vi "main.vi"() -> ()   [LabVIEW 2016]
uses:
  <vilib>/myRIO/Instrument Drivers/Onboard IO/DIO/typedefs/DIO Reference.ctl
  <vilib>/myRIO/Common/Instrument Driver Framework/Utilities/typedefs/myRIO Generic Hardware Reference.ctl
  <vilib>/myRIO/Common/Instrument Driver Framework/Utilities/typedefs/Hardware Version Enum.ctl
  <vilib>/myRIO/Common/Instrument Driver Framework/Utilities/typedefs/myRIO v1.0 Reference.ctl
  <vilib>/myRIO/Common/Instrument Driver Framework/Utilities/typedefs/Generic FPGA Reference.ctl
  <vilib>/myRIO/Common/Instrument Driver Framework/myRIO v1.0/DIO/typedefs/DIO Channels List.ctl
  <vilib>/myRIO/Common/Instrument Driver Framework/myRIO v1.0/DIO/typedefs/DIO Channels Enum.ctl
  <vilib>/userdefined/High Color/nirio_resource_hc.ctl
  <vilib>/userdefined/High Color/IMAQdx.ctl
  <vilib>/vision/Instrument.llb/QR Code Search Options.ctl
  <vilib>/vision/Instrument.llb/Demodulation Mode.ctl
  <vilib>/vision/Instrument.llb/Cell Sample Size.ctl
  <vilib>/vision/Instrument.llb/Cell Filter Mode.ctl
  <vilib>/vision/driver/IMAQdx.llb/IMAQdx Camera Control Mode.ctl
  <vilib>/myRIO/Common/Instrument Driver Framework/Utilities/vis/Is FPGA Ref Available.vi
  <vilib>/myRIO/Common/Instrument Driver Framework/myRIO v1.0/DIO/vis/myRIO v1.1 Open DIO.vi
  <vilib>/myRIO/Instrument Drivers/Onboard IO/DIO/vis/Write.vi
  <vilib>/myRIO/Instrument Drivers/Onboard IO/DIO/vis/Read.vi
  <vilib>/myRIO/Common/Instrument Driver Framework/Utilities/vis/Validate Channels.vi
  <vilib>/myRIO/Common/Instrument Driver Framework/myRIO v1.0/DIO/vis/myRIO v1.0 Reserve DIO.vi
  <vilib>/myRIO/Common/Instrument Driver Framework/myRIO v1.0/UART/vis/myRIO v1.0 Close UART.vi
  <vilib>/myRIO/Common/Instrument Driver Framework/myRIO v1.0/Resource Manager/vis/myRIO v1.0 Reserve Channel List.vi
  <vilib>/myRIO/Common/Instrument Driver Framework/myRIO v1.0/DIO/vis/myRIO v1.0 Build MUX Configuration DIO.vi
  <vilib>/myRIO/Common/Instrument Driver Framework/myRIO v1.0/Resource Manager/vis/myRIO v1.0 Reserve Channel.vi
  <vilib>/myRIO/Common/Instrument Driver Framework/myRIO v1.0/Resource Manager/vis/myRIO v1.0 Unreserve Channel.vi
  <vilib>/myRIO/Common/Instrument Driver Framework/myRIO v1.0/Resource Manager/vis/myRIO v1.0 Create Configuration List.vi
  <vilib>/myRIO/Common/Instrument Driver Framework/myRIO v1.0/Resource Manager/vis/myRIO v1.0 Build Mutex Name.vi
  <vilib>/Utility/VariantDataType/GetNumericInfo.vi
  <vilib>/Utility/error.llb/Error Cluster From Error Code.vi
  <vilib>/myRIO/Common/Instrument Driver Framework/myRIO v1.0/myRIO v1.1 Open.vi
  <vilib>/myRIO/Common/Instrument Driver Framework/Utilities/vis/IO Manager.vi
  <vilib>/myRIO/Common/Instrument Driver Framework/Utilities/vis/Configuration Manager.vi
  <vilib>/myRIO/Common/Instrument Driver Framework/myRIO v1.0/Resource Manager/vis/myRIO v1.0 Configure IO.vi
  <vilib>/myRIO/Common/Instrument Driver Framework/myRIO v1.0/myRIO v1.0 Close.vi
  <vilib>/myRIO/Common/Instrument Driver Framework/myRIO v1.0/DIO/vis/myRIO v1.0 Write DIO.vi
  <vilib>/myRIO/Common/Instrument Driver Framework/myRIO v1.0/DIO/vis/myRIO v1.0 Read DIO.vi
  <vilib>/Utility/file.llb/Read Delimited Spreadsheet (string).vi
  <vilib>/myRIO/Common/Instrument Driver Framework/Utilities/vis/FPGA Ref Manager.vi
  <vilib>/myRIO/Common/Instrument Driver Framework/myRIO v1.0/myRIO v1.0 Reset FPGA.vi
  <vilib>/myRIO/Common/Instrument Driver Framework/myRIO v1.0/IRQ/vis/myRIO v1.0 IRQ Info FGV.vi
  <vilib>/myRIO/Common/Instrument Driver Framework/myRIO v1.0/IRQ/vis/myRIO v1.0 Timer IRQ Info FGV.vi
  <vilib>/myRIO/Common/Instrument Driver Framework/myRIO v1.0/IRQ/vis/myRIO v1.0 ISR Agent.vi
  <instrlib>/Hokuyo URG Series/Public/Initialize-cRIO-USB.vi
  <vilib>/myRIO/Express VI/Onboard Devices/LED/LED Express VI.xnode
  <vilib>/myRIO/Instrument Drivers/Onboard IO/DIO/vis/myRIO DIO Open.xnode
  <vilib>/myRIO/Express VI/Onboard IO/DI/DI Express VI.xnode
  <vilib>/myRIO/Instrument Drivers/Onboard IO/DIO/DIO.lvlib
  <vilib>/vision/driver/NI_Vision_Acquisition_Software.lvlib
  <vilib>/myRIO/Instrument Drivers/Utilities/Utilities.lvlib
  <instrlib>/Hokuyo URG Series/Hokuyo URG Series.lvlib
  <vilib>/vision/NI_Vision_Development_Module.lvlib
panel:
  out "Color Footage":T1(plugin-control)
  out "QR Footage":T1(plugin-control)
  out "QR Attempts":i32
  out "Data":string
  out "?":errorcluster
  out "Algorithm log":string
  out "Cubes 3 Flag":bool
  out "Delete Files":bool
  out "Hokuyo Init":bool
  out "hokuyo instance":dbl[](array[numeric])
  out "hokuyo":dbl[](array[numeric])
  out "COLOR CUBE":dbl
  out "COLOR BOX":dbl
  out "Box Array":dbl[](array[numeric])
  out "Cube Array":dbl[](array[numeric])
  out "Box Green":dbl
  out "Box Red":dbl
  out "Box Blue":dbl
  out "Cube Green":dbl
  out "Cube Red":dbl
  out "Cube Blue":dbl
  out "Colors String":string
  out "QR BREAK":bool
  out "CHECK route2.csv":bool
  out "Route Size Array":dbl[](array[numeric])
  out "MovementCounter":dbl
  out "ActionCounter":dbl
  out "Route Size":dbl
  out "Action":dbl
  out "Movement":dbl
  out "Route":string[][](array[string])
  out "START ALGO":bool
  out "CHECK route1.csv":bool
  out "TERMINAL OUTPUT":string
  out "STD ERROR":string
  out "RETURN VALUE":i32
  # "+\n+\n+\n+\n+\n+\n+\n+\n+\n+\n+\n+\n+\n+\n+\n+\n+\n+\n+\n+\n+\n+\n+\n+\n+\n+\n+\n+\n+\n+\n+\n+\n+\n+\n+\n+\n+\n+\n+\n+\n+\n+\n+\n+\n+\n+\n+\n+\n+\n+\n+\n+\n+\n+\n+\n+\n+\n+\n+\n+\n+"
  # "+\n+\n+\n+\n+\n+\n+\n+\n+\n+\n+\n+\n+\n+\n+\n+\n+\n+\n+\n+\n+"
  # "++++++++++++++++++++++++++++++++++++++++++++++++++++++++++++++++++++++++++++++++++++++++++++++++++++++++++++++++++++++++++++++++++++++++++++++++++++++++++++++++++++++++++++++++++++++++++++++++++++++++++++++++++++++++++++++++++++++++"
  # "+\n+\n+\n+\n+\n+\n+\n+\n+\n+\n+\n+\n+\n+\n+\n+\n+\n+\n+\n+\n+\n+\n+\n+\n+\n+\n+\n+\n+\n+\n+\n+\n+\n+\n+\n+\n+\n+\n+\n+\n+\n+\n+\n+\n+\n+\n+\n+\n+\n+\n+\n+\n+\n+\n+\n+\n+\n+\n+\n+"
  # "+\n+\n+\n+\n+\n+\n+\n+\n+\n+\n+\n+\n+\n+\n+\n+\n+\n+\n+\n+\n+\n+\n+\n+\n+\n+\n+\n+\n+\n+\n+\n+\n+\n+\n+\n+\n+\n+\n+\n+\n+\n+\n+\n+\n+\n+\n+\n+"
  # "+\n+\n+\n+\n+\n+\n+\n+\n+\n+\n+\n+\n+\n+\n+\n+\n+\n+\n+\n+\n+"
  # "+\n+\n+\n+\n+\n+\n+\n+\n+\n+\n+\n+\n+\n+\n+\n+\n+\n+\n+\n+\n+"
  # "INDICATORS"
  # "QR INDICATOR"
  # "ALGORITHM"
  # "NUMERIC INDICATORS"
  # "INFO"
  # "Actions:\n\n0) Finish\n1) Front\n2) Back\n3) Right\n4) Left\n5) Calibrate\n6) Take and Store\n7) Take and Hold\n8) Place cube\n9) Color Check\n10) Park\n15) No Calibration"
  # "Colors:\n\n10) Blue\n11) Green\n12) Yellow\n13) Red\n14) Orange\n15) Unknown"
  # "++++++++++++++++++++++++++++++++++++++++++++++++++++++++++++++++++++++++++++++++++++++++++++++++++++++++++++++++++++++++++++++++++++++++++++++++++++++++++++++++++++++++++++++++++++++++++++++++++++++++++++++++++++++++++++++++++++++"
  # "+\n+\n+\n+\n+\n+\n+\n+\n+\n+\n+\n+\n+\n+\n+\n+\n+\n+\n+\n+\n+\n+\n+\n+\n+\n+"
  # "+\n+\n+\n+\n+\n+\n+\n+\n+\n+\n+\n+\n+\n+\n+\n+\n+\n+\n+\n+\n+\n+\n+\n+\n+\n+\n+\n+\n+\n+\n+\n+\n+\n+\n+\n+\n+\n+"
  # "BASH CLEANUP SCRIPT"
  # "ROUTE FILES CHECK"
  # "ROUTE READING"
  # "++++++++++++++++++++++++++++++++++++++++++++++++++++++++++++++++++++++++++++++++++++++++++++++++++++++++++++++++"
  # "HOKUYO CALIBRATION"
  # "10"
  # "11"
  # "++++++++++++++++++++++++++++++++++++++++++++++++++++++++++++++++++++++++++++++++++++++++++++++++++++++++++++++++++++++++++++++++++++++++++++++++++++++++++++++++++++++++++++++++++++++++++++++++++++++++++++++++++++++++++++++++++++++++"
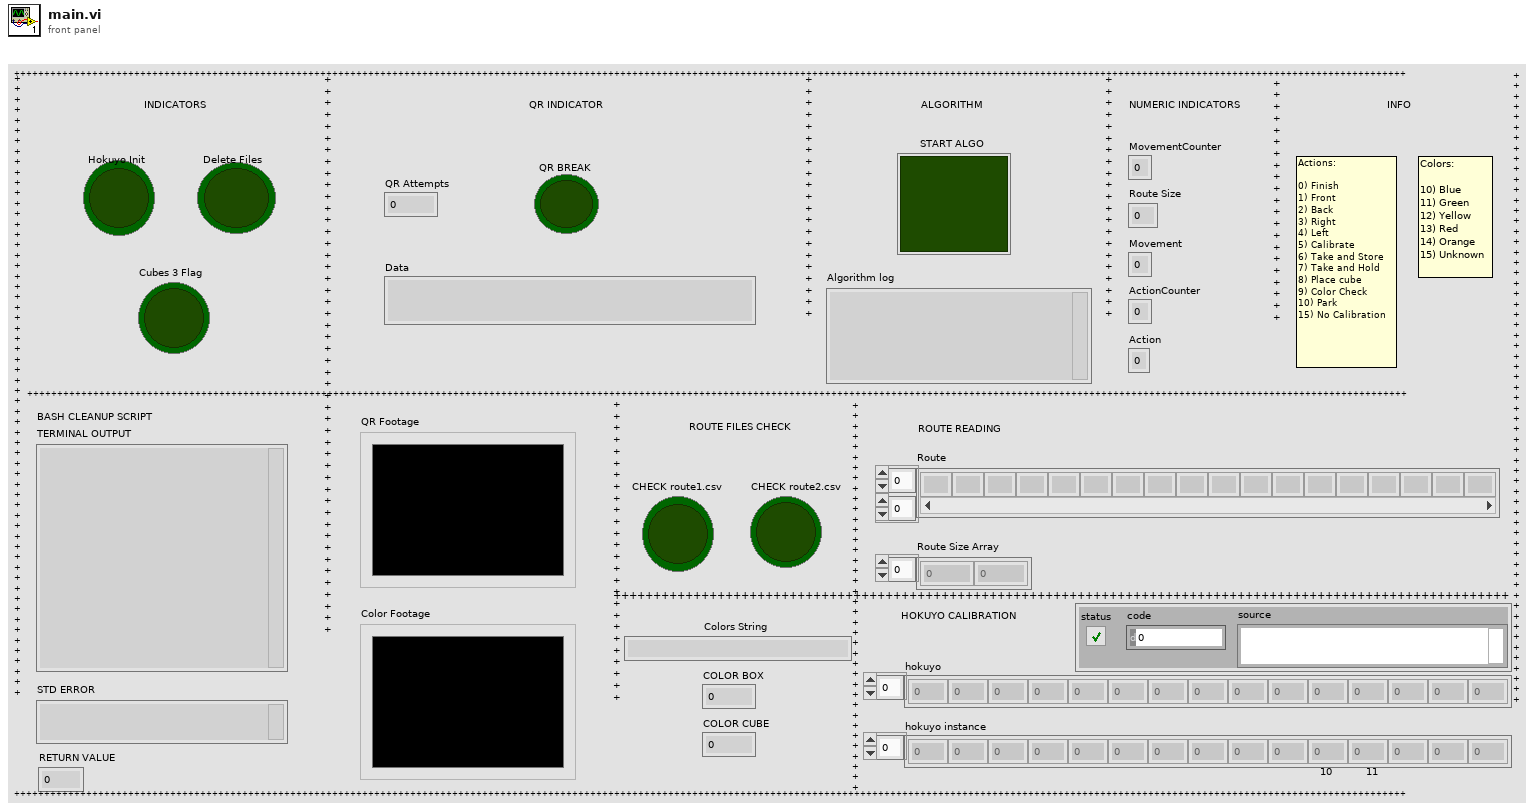
[diagram p1: front panel]
types:
  T1 = typedef "IMAQ Image.ctl" = refnum<image>
  T2 = typedef "DIO.lvlib/DIO Reference.ctl" = cluster{"myRIO Reference":T3, "DIO Channels List":T7}
  T3 = typedef "myRIO Generic Hardware Reference.ctl" = cluster{"myRIO Model":T4, "myRIO Hardware Reference":T5}
  T4 = typedef "Hardware Version Enum.ctl" = enum16{"Unknown", "myRIO-1900", "myRIO-1950", "roboRIO", "NI ELVIS RIO CM"}
  T5 = typedef "myRIO v1.0 Reference.ctl" = cluster{"Generic FPGA Reference":T6, "Allow multiple opens":bool}
  T6 = typedef "Generic FPGA Reference.ctl" = refnum<k20>
  T7 = typedef "DIO Channels List.ctl" = T8[]
  T8 = typedef "DIO Channels Enum.ctl" = enum16{"Not Connected", "C/DIO0", "C/DIO1", "C/DIO2", "C/DIO3", "C/DIO4", "C/DIO5", "C/DIO6", "C/DIO7", "A/DIO0", "A/DIO1", "A/DIO2", "A/DIO3", "A/DIO4", "A/DIO5", "A/DIO6", "A/DIO7", "A/DIO8", "A/DIO9", "A/DIO10", "A/DIO11", "A/DIO12", "A/DIO13", "A/DIO14", "A/DIO15", "B/DIO0", "B/DIO1", "B/DIO2", "B/DIO3", "B/DIO4", "B/DIO5", "B/DIO6", "B/DIO7", "B/DIO8", "B/DIO9", "B/DIO10", "B/DIO11", "B/DIO12", "B/DIO13", "B/DIO14", "B/DIO15", "LED0", "LED1", "LED2", "LED3", "Button0", "DIO/DIO0", "DIO/DIO1", "DIO/DIO2", "DIO/DIO3", "DIO/DIO4", "DIO/DIO5", "DIO/DIO6", "DIO/DIO7", "DIO/DIO8", "DIO/DIO9", "SPI/CS0", "SPI/CS1", "SPI/CS2", "SPI/CS3", "LED RADIO (Green)", "LED RADIO (Red)", "LED COMM (Green)", "LED COMM (Red)", "LED MODE (Green)", "LED MODE (Red)"}
  T9 = typedef "nirio_resource_hc.ctl" = tag
  T10 = typedef "IMAQdx.ctl" = refnum<k21>
  T11 = typedef "QR Code Search Options.ctl" = cluster{"Rotation Mode":enum32{"Unlimited", "0 Degrees", "90 Degrees", "180 Degrees", "270 Degrees"}, "Skip Location?":bool, "Edge Threshold":u32, "Demodulation Mode":T12, "Cell Sample Size":T13, "Cell Filter Mode":T14, "Skew Degrees Allowed":u32}
  T12 = typedef "Demodulation Mode.ctl" = i32
  T13 = typedef "Cell Sample Size.ctl" = i32
  T14 = typedef "Cell Filter Mode.ctl" = i32
  T15 = typedef "NI_Vision_Acquisition_Software.lvlib/IMAQdx Camera Control Mode.ctl" = enum32{"Controller", "Listener"}
  T16 = typedef "Image Type" = u32
  T17 = typedef "QR Code Report.ctl" = cluster{"Found?":bool, "Data":string, "Bounding Box":cluster{"x":sgl, "y":sgl}[], "Errors Corrected":u32, "Dimensions (Rows/Cols)":u32, "Version":u32, "QR Model":T18, "Stream Mode":T19, "Barcode Polarity":T20, "Mirrored?":bool, "Append Stream Position":u32, "Size of Append Stream":u32, "First EAN-128 ID":i32, "First Alternate Language ID":i32, "Append Stream ID":u32, "Minimum Edge Strength":u32, "Demodulation Mode":T12, "Cell Sample Size":T13, "Cell Filter Mode":T14}
  T18 = typedef "QR Code Model Type.ctl" = i32
  T19 = typedef "QR Code Stream Mode Type.ctl" = i32
  T20 = typedef "Data Matrix Polarity.ctl" = i32
  T21 = cluster{"histogram":u32[], "Minimal Value":sgl, "Maximal Value":sgl, "Starting Value":sgl, "Interval Width":sgl, "Mean Value":sgl, "Standard  Variation":sgl, "Area (pixels)":i32}
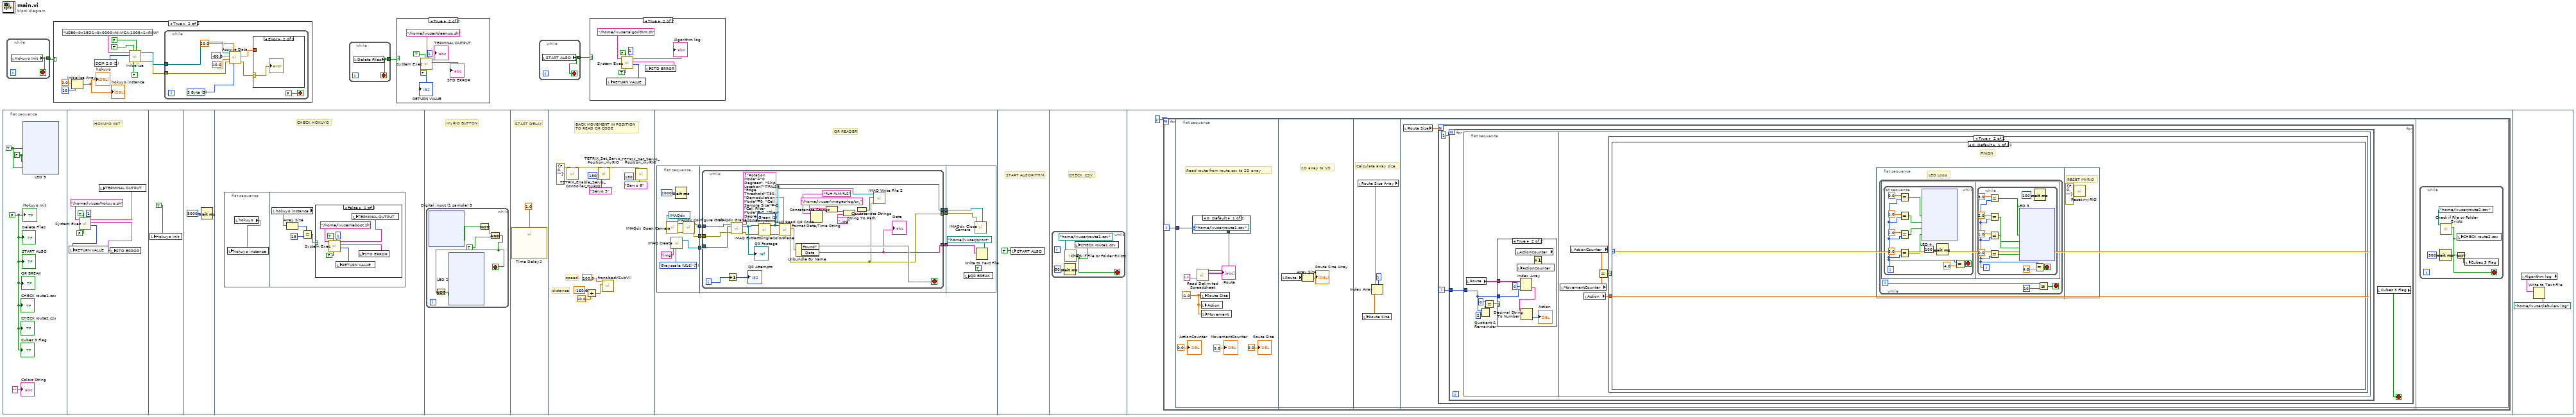
[diagram p0: block diagram]
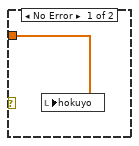
[diagram p4: hidden frame]
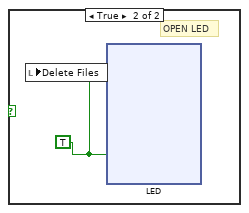
[diagram p6: hidden frame]
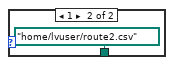
[diagram p7: hidden frame]
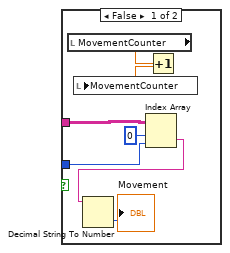
[diagram p8: hidden frame]
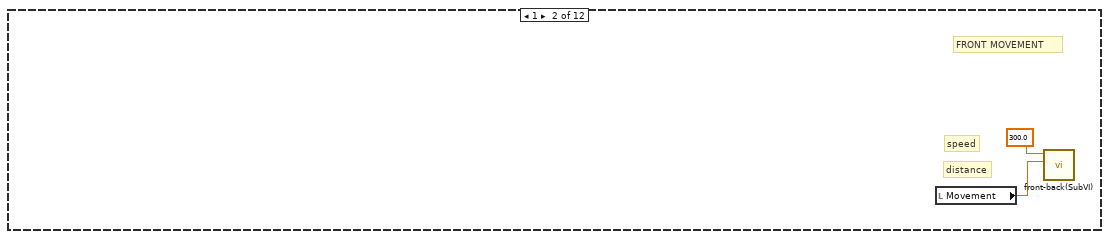
[diagram p10: hidden frame]
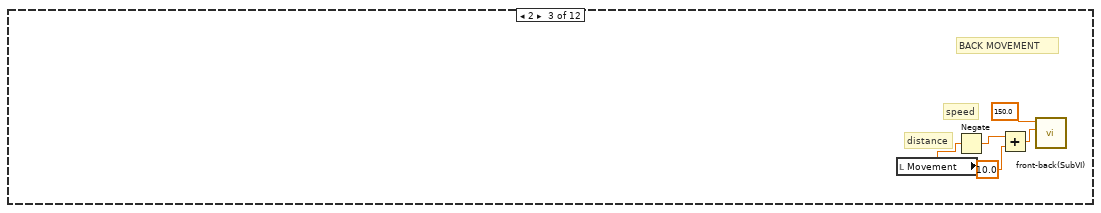
[diagram p11: hidden frame]
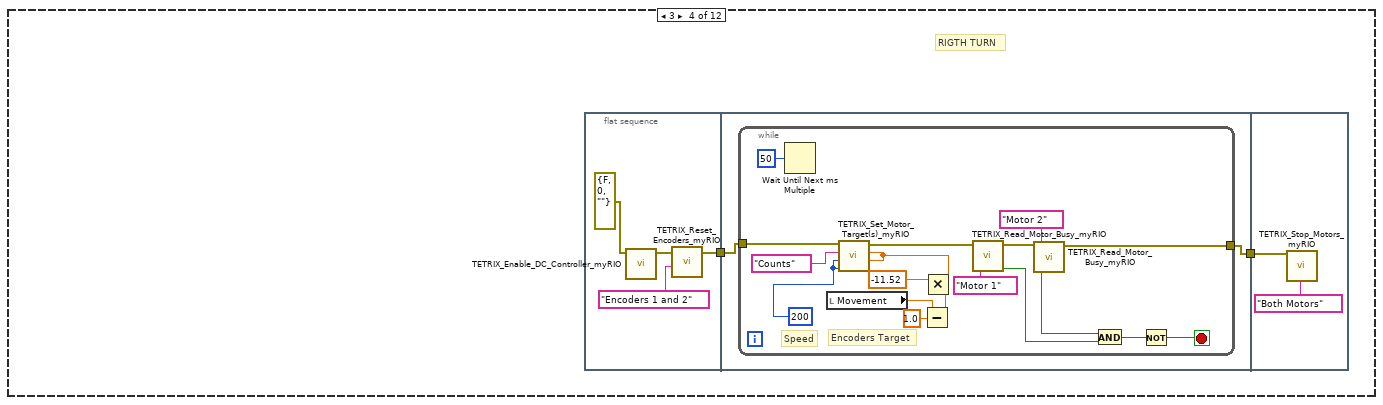
[diagram p12: hidden frame]
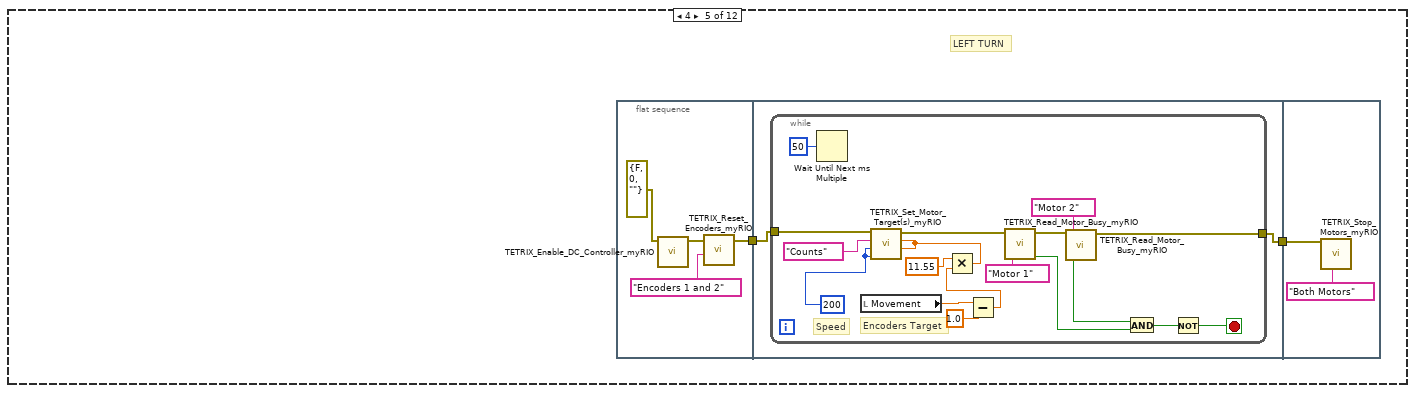
[diagram p13: hidden frame]
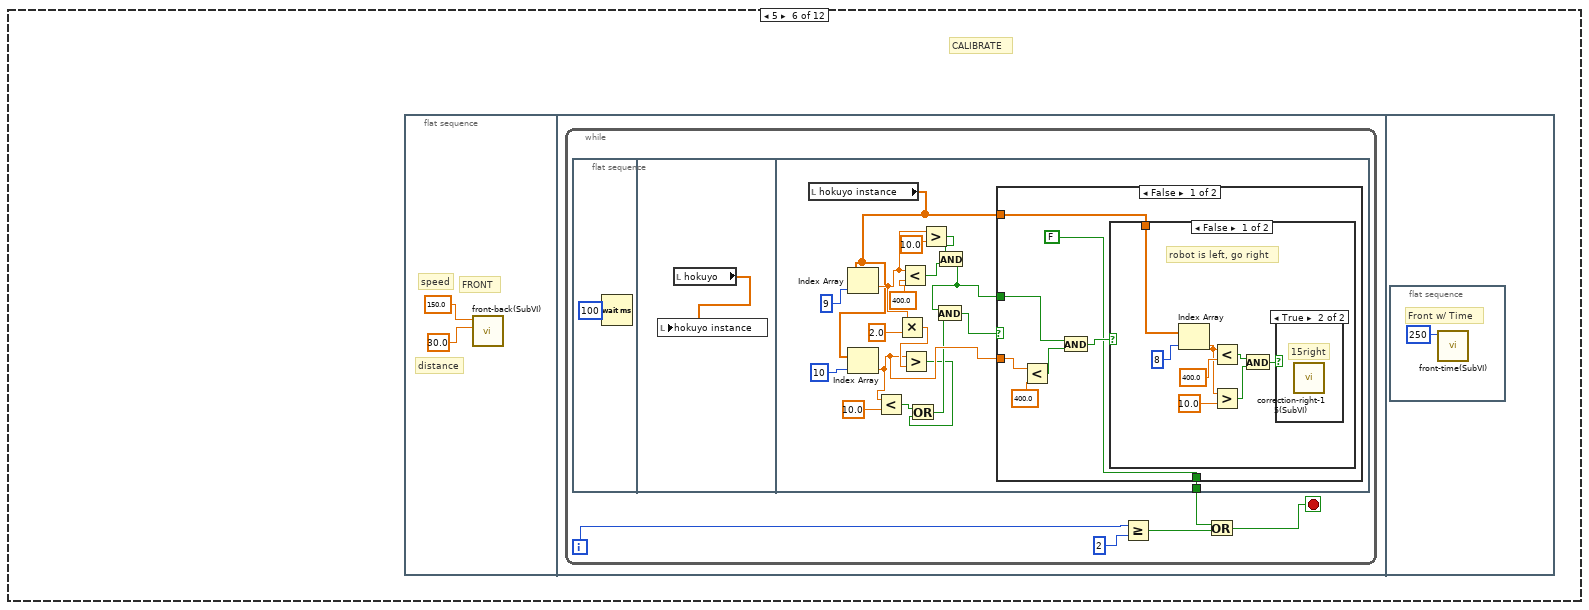
[diagram p14: hidden frame]
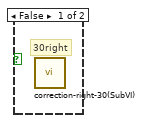
[diagram p15: hidden frame]
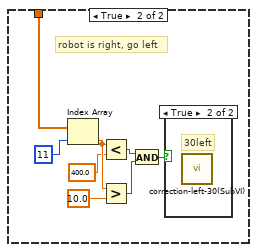
[diagram p16: hidden frame]
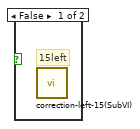
[diagram p17: hidden frame]
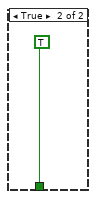
[diagram p18: hidden frame]
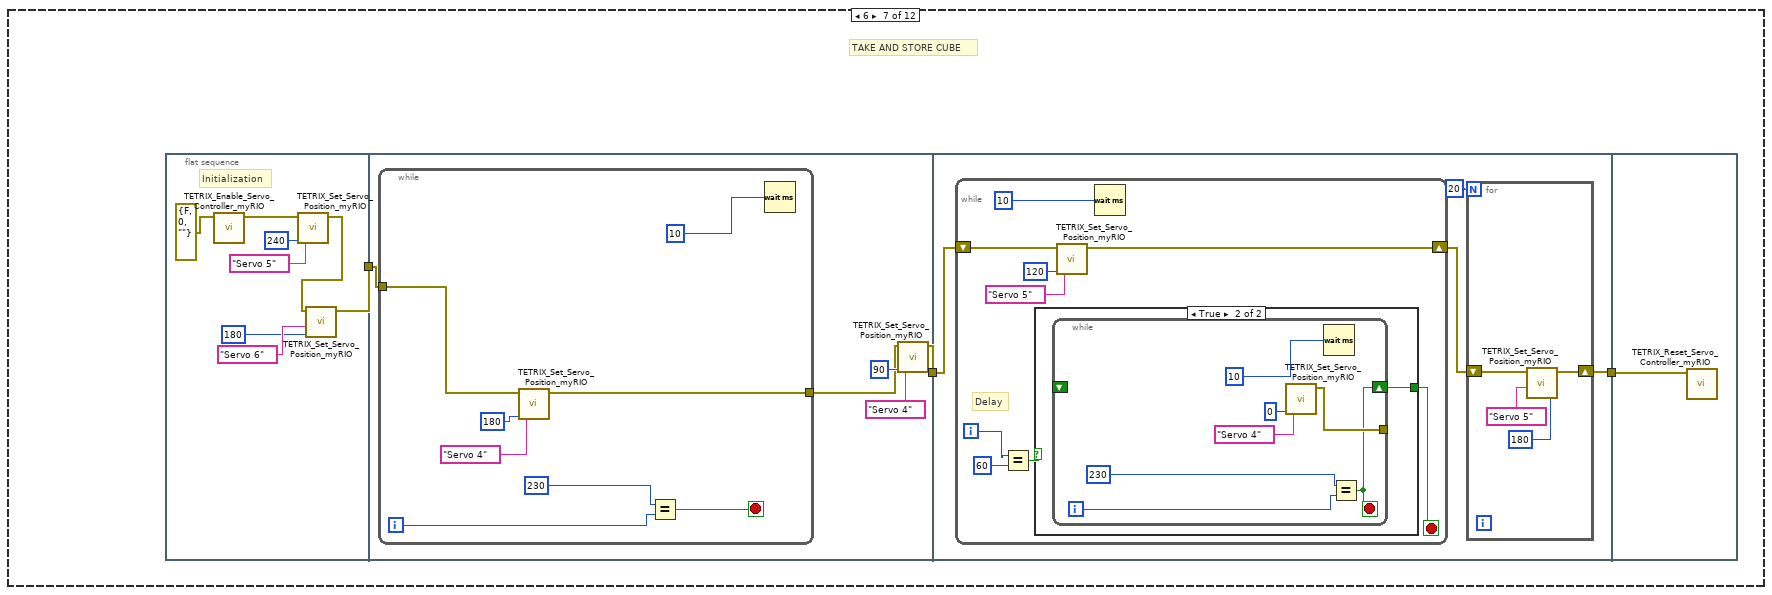
[diagram p19: hidden frame]
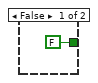
[diagram p20: hidden frame]
diagram:
  n1 = flat-sequence {
    frame #0 {
      w4 = FALSE ("START ALGO")
      w6 = FALSE ("LED1")
      w5 = TRUE ("LED0")
      n2 = xnode "LED 5"("LED0"=w5, "LED1"=w6, "LED2"=w6, "LED3"=w5) -> ()  [unwired: 1 in, 1 out]
      "START ALGO" <- w4
      "QR BREAK" <- w4
      "CHECK route2.csv" <- w4
      "CHECK route1.csv" <- w4
      "Colors String" <- "" ("Colors String")
      "Delete Files" <- w4
      "Hokuyo Init" <- w4
      "Cubes 3 Flag" <- w4
    }
    frame #1 {
      # "HOKUYO INIT"
      n3 = call <vilib>:"System Exec.vi"("expected output size  (4096)"=u32 1, "run minimized? (F)"=FALSE, "wait until completion? (T)"=TRUE, "command line"="/home/lvuser/hokuyo.sh") -> ("return code"=w52:i32, "standard error"=w51:string, "standard output"=w50:string)  [unwired: 4 in, 1 out]
      n4 = local write "RETURN VALUE"(w52) -> ()
      n5 = local write "TERMINAL OUTPUT"(w50) -> ()
      n6 = local write "STD ERROR"(w51) -> ()
    }
    frame #2 {
      n7 = local write "Hokuyo Init"(TRUE) -> ()
    }
    frame #3 {
      n8 = Wait (ms)(milliseconds to wait=u32 5000) -> ()  [unwired: 1 out]
    }
    frame #4 {
      # "CHECK HOKUYO"
      n9 = flat-sequence {
        frame #0 {
          n10 = local read "hokuyo"() -> (w55:dbl[])
          n11 = local write "hokuyo instance"(w55) -> ()
        }
        frame #1 {
          n12 = local read "hokuyo instance"() -> (w56:dbl[])
          n13 = Array Size(array=w56) -> (size(s)=w57:i32)
          n14 = Equal?(x=w57, y=15) -> (x = y?=w58:bool)
          n15 = case shown="False" w58 {
            frame False {
              n16 = call <vilib>:"System Exec.vi"("expected output size  (4096)"=u32 1, "run minimized? (F)"=FALSE, "wait until completion? (T)"=TRUE, "command line"="/home/lvuser/reboot.sh") -> ("return code"=w62:i32, "standard error"=w61:string, "standard output"=w60:string)  [unwired: 4 in, 1 out]
              n17 = local write "RETURN VALUE"(w62) -> ()
              n18 = local write "TERMINAL OUTPUT"(w60) -> ()
              n19 = local write "STD ERROR"(w61) -> ()
            }
            frame True {
              w67 = TRUE ("LED0")
              # "OPEN LED"
              n20 = local write "Delete Files"(w67) -> ()
              n21 = xnode "LED"("LED0"=w67, "LED1"=w67, "LED2"=w67, "LED3"=w67) -> ()  [unwired: 1 in, 1 out]
            }
          }
        }
      }
    }
    frame #5 {
      # "myRIO BUTTON"
      n22 = while {
        stop <- w108 stop-if-true
        n23 = xnode "Digital input (1 sample) 3"() -> ("A/DIO13 (Pin 26)"=w107:bool)  [unwired: 1 in, 1 out]
        n24 = Not(x=w107) -> (.not. x?=w106:bool)
        n25 = And(x=w106, y=TRUE) -> (x .and. y?=w108:bool)
        n26 = Not(x=w108) -> (.not. x?=w110:bool)
        n27 = xnode "LED 2"("LED0"=w110, "LED1"=w110, "LED2"=w110, "LED3"=w110) -> ()  [unwired: 1 in, 1 out]
      }
    }
    frame #6 {
      # "START DELAY"
      n28 = call "Time Delay2"("Delay Time (s)"=1.0) -> ()  [unwired: 10 in, 1 out]
    }
    frame #7 {
      # "speed"
      # "distance"
      # "BACK MOVEMENT IN POSITION\nTO READ QR CODE"
      n29 = call <vilib>:"TETRIX_Enable_Servo_Controller_myRIO.vi"("Error/Flow In"=errorcluster {"status"=FALSE, "code"=0, "source"=""}) -> ("Error/Flow Out"=w194:errorcluster)  [unwired: 6 in]
      n30 = Add(x=-160.0 ("distance"), y=10.0) -> (x+y=w185:dbl)
      n31 = call <vilib>:"TETRIX_Set_Servo_Position_myRIO.vi"("Set Servo Position (0 - 180 degrees)"=u8 180, "Select Channel"="Servo 5", "Error/Flow In"=w194) -> ("Error/Flow Out"=w189:errorcluster)  [unwired: 4 in]
      n32 = call "front-back(SubVI).vi"("distance"=w185, "speed"=100.0) -> ()  [unwired: 10 in]
      n33 = call <vilib>:"TETRIX_Set_Servo_Position_myRIO.vi"("Set Servo Position (0 - 180 degrees)"=u8 180, "Select Channel"="Servo 6", "Error/Flow In"=w189) -> ()  [unwired: 4 in, 1 out]
    }
    frame #8 {
      # "QR READER"
      n34 = flat-sequence {
        tunnel: [w209] -> w201
        tunnel: [w204] -> w197
        tunnel: [w203] -> w196
        tunnel: w201 -> [w215]
        tunnel: [w214] -> w200
        tunnel: [w216] -> w199
        tunnel: [w213] -> w198
        tunnel: w197 -> [w212]
        tunnel: w196 -> [w211]
        tunnel: w200 -> [w240]
        tunnel: w199 -> [w241]
        tunnel: w198 -> [w242]
        frame #0 {
          w207 = T16 7 items=["Grayscale (U8)", "Grayscale (I16)", "Grayscale (SGL)", "Complex (CSG)", "RGB (U32)", "HSL (U32)", "RGB (U64)", "Grayscale (U16)"] ("Image Type")
          n35 = call <vilib>:"IMAQdx Open Camera.vi"("Session In"=T10 "cam0") -> ("error out"=w205:errorcluster, "Session Out"=w206:T10)  [unwired: 9 in]
          n36 = call "IMAQ Create"("Image Name"="img", "Image Type"=w207) -> ("New Image"=w209:T1)  [unwired: 3 in, 1 out]
          n37 = Wait (ms)(milliseconds to wait=u32 2000) -> ()  [unwired: 1 out]
          n38 = call <vilib>:"IMAQdx Configure Grab.vi"("error in"=w205, "Session In"=w206) -> ("error out"=w203:errorcluster, "Session Out"=w204:T10)  [unwired: 8 in]
        }
        frame #1 {
          n39 = while {
            tunnel: [w221] -> w216
            tunnel: [w217] -> w214
            tunnel: w215 -> [w239]
            tunnel: [w233] -> w213
            tunnel: w212 -> [w229]
            tunnel: w211 -> [w228]
            i -> [w232]
            stop <- w235 stop-if-true
            w238 = 1 items=["Red", "Green", "Blue", "Hue", "Saturation", "Luminance", "Value", "Intensity"] ("Color Plane")
            n40 = Increment(x=w232) -> (x+1=→"QR Attempts":i32)
            n41 = call <vilib>:"IMAQdx Grab2.vi"("error in"=w228, "Image In"=w239, "Session In"=w229) -> ("error out"=w234:errorcluster, "Image Out"=w230:T1, "Session Out"=w221:T10)  [unwired: 5 in, 1 out]
            "QR Footage" <- w230
            n42 = call "IMAQ ExtractSingleColorPlane"("Color Plane"=w238, "error in (no error)"=w234, "Image Src"=w230) -> ("error out"=w237:errorcluster, "Image Dst Out"=w220:T1)  [unwired: 7 in]
            n43 = call "IMAQ Read QR Code"("QR Search Options"=T11 {"Rotation Mode"=enum."0 Degrees", "Skip Location?"=FALSE, "Edge Threshold"=30, "Demodulation Mode"=0, "Cell Sample Size"=-2, "Cell Filter Mode"=-2, "Skew Degrees Allowed"=5}, "error in (no error)"=w237, "Image"=w220) -> ("error out"=w217:errorcluster, "QR Code Report"=w236:T17)  [unwired: 5 in, 2 out]
            n44 = Unbundle By Name(w236) -> ("Found?"=w235:bool, "Data"=w233:string)
            "Data" <- w233
            n45 = Format Date/Time String(time format string (%c)="%H-%M-%S") -> (date/time string=w227:string)  [unwired: 2 in]
            n46 = Concatenate Strings("/home/lvuser/images-log/qr_" ("string"), w227) -> (w225:string)
            n47 = Concatenate Strings(w225, ".jpg" ("string")) -> (w222:string)
            n48 = String To Path(string=w222) -> (path=w219:path)
            n49 = call-poly "IMAQ Write File 2"("error in (no error)"=w217, "File Path"=w219, "Image"=w220) -> ()  [unwired: 7 in, 2 out]
          }
        }
        frame #2 {
          n50 = local write "QR BREAK"(TRUE ("QR BREAK")) -> ()
          n51 = call <vilib>:"IMAQdx Close Camera.vi"("error in"=w240, "Session In"=w241) -> ()  [unwired: 9 in, 1 out]
          n52 = Write to Text File(file (use dialog)=path "/home/lvuser/qr.txt", text=w242) -> ()  [unwired: 2 in, 3 out]
        }
      }
    }
    frame #9 {
      # "START ALGORITHM"
      n53 = local write "START ALGO"(TRUE ("START ALGO")) -> ()
    }
    frame #10 {
      # "CHECK .CSV"
      n54 = while {
        stop <- w246 stop-if-true
        n55 = Wait (ms)(milliseconds to wait=u32 50) -> ()  [unwired: 1 out]
        n56 = call <vilib>:"Check if File or Folder Exists.vi"("path"=path "/home/lvuser/route1.csv" ("file (use dialog)")) -> ("file or folder exists?"=w246:bool)  [unwired: 8 in, 2 out]
        n57 = local write "CHECK route1.csv"(w246) -> ()
      }
    }
    frame #11 {
      n58 = for {
        N: 2 -> [_]
        i -> [w250]
        n59 = flat-sequence {
          tunnel: w250 -> [w258]
          frame #0 {
            w254 = -1.0 ("Route Size")
            # "Read route from route.csv to 2D array"
            n60 = case shown="0, Default" w258 {
              tunnel: [path "/home/lvuser/route1.csv" ("file (use dialog)") path "/home/lvuser/route2.csv" ("file (use dialog)")] -> w255
              frame 0, Default {
              }
              frame 1 {
              }
            }
            n61 = call-poly <vilib>:"Read Delimited Spreadsheet.vi"("file path (dialog if empty)"=w255, "delimiter (\\t)"="," ("delimiter (\\t)")) -> ("all rows"=→"Route":string[][])  [unwired: 8 in, 5 out]
            n62 = local write "Route Size"(w254) -> ()
            n63 = local write "Action"(w254) -> ()
            n64 = local write "Movement"(w254) -> ()
            "ActionCounter" <- 0.0 ("ActionCounter")
            "MovementCounter" <- 0.0 ("MovementCounter")
            "Route Size" <- 0.0 ("Route Size")
          }
          frame #1 {
            # "2D array to 1D"
            n65 = local read "Route"() -> (w261:string[][])
            n66 = Array Size(array=w261) -> (size(s)=→"Route Size Array":i32[])
          }
          frame #2 {
            # "Calculate array size"
            n67 = local read "Route Size Array"() -> (w264:dbl[])
            n68 = Index Array(array=w264, index=1) -> (element=w263:dbl)
            n69 = local write "Route Size"(w263) -> ()
          }
          frame #3 {
            n70 = local read "Route Size"() -> (w266:dbl)
            n71 = for {
              N: w266 -> [_]
              i -> [w269]
              stop <- w267 stop-if-true
              n72 = for {
                N: 1 -> [_]
                tunnel: w269 -> [w270]
                n73 = flat-sequence {
                  tunnel: w270 -> [w273]
                  frame #0 {
                    n74 = local read "Route"() -> (w271:string[][])
                    n75 = Quotient & Remainder(x=w273, y=2) -> (x-y*floor(x/y)=w275:i32)  [unwired: 1 out]
                    n76 = Equal?(x=0, y=w275) -> (x = y?=w272:bool)
                    n77 = case shown="True" w272 {
                      tunnel: w273 -> [w280 w288]
                      tunnel: w271 -> [w281 w286]
                      frame False {
                        n78 = local read "MovementCounter"() -> (w278:dbl)
                        n79 = Index Array(array=w281, index (row)=0, index (col)=w280) -> (element=w282:string)
                        n80 = Decimal String To Number(string=w282) -> (number=→"Movement":i32)  [unwired: 2 in, 1 out]
                        n81 = Increment(x=w278) -> (x+1=w277:dbl)
                        n82 = local write "MovementCounter"(w277) -> ()
                      }
                      frame True {
                        n83 = local read "ActionCounter"() -> (w290:dbl)
                        n84 = Index Array(array=w286, index (row)=0, index (col)=w288) -> (element=w285:string)
                        n85 = Decimal String To Number(string=w285) -> (number=→"Action":i32)  [unwired: 2 in, 1 out]
                        n86 = Increment(x=w290) -> (x+1=w289:dbl)
                        n87 = local write "ActionCounter"(w289) -> ()
                      }
                    }
                  }
                  frame #1 {
                    n88 = local read "MovementCounter"() -> (w292:dbl)
                    n89 = local read "ActionCounter"() -> (w293:dbl)
                    n90 = local read "Action"() -> (w291:dbl)
                    n91 = Equal?(x=w293, y=w292) -> (x = y?=w294:bool)
                    n92 = case shown="True" w294 {
                      tunnel: w291 -> [_ w295]
                      frame False {
                      }
                      frame True {
                        n93 = case shown="0, Default" w295 {
                          frame 0, Default {
                            # "FINISH"
                            n94 = flat-sequence {
                              frame #0 {
                                # "LED Loop"
                                n95 = while {
                                i -> [w297]
                                stop <- w298 stop-if-true
                                n96 = flat-sequence {
                                frame #0 {
                                n97 = while {
                                i -> [w301]
                                stop <- w300 stop-if-true
                                n98 = Equal?(x=0.0, y=w301) -> (x = y?=w306:bool)
                                n99 = Equal?(x=1.0, y=w301) -> (x = y?=w305:bool)
                                n100 = Equal?(x=2.0, y=w301) -> (x = y?=w304:bool)
                                n101 = Equal?(x=3.0, y=w301) -> (x = y?=w303:bool)
                                n102 = xnode "LED 4"("LED0"=w306, "LED1"=w305, "LED2"=w304, "LED3"=w303) -> ()  [unwired: 1 in, 1 out]
                                n103 = Wait (ms)(milliseconds to wait=u32 100) -> ()  [unwired: 1 out]
                                n104 = Equal?(x=w301, y=4.0) -> (x = y?=w300:bool)
                                }
                                }
                                frame #1 {
                                n105 = while {
                                i -> [w351]
                                stop <- w350 stop-if-true
                                n106 = Equal?(x=3.0, y=w351) -> (x = y?=w356:bool)
                                n107 = Equal?(x=2.0, y=w351) -> (x = y?=w355:bool)
                                n108 = Equal?(x=1.0, y=w351) -> (x = y?=w354:bool)
                                n109 = Equal?(x=0.0, y=w351) -> (x = y?=w353:bool)
                                n110 = xnode "LED 3"("LED0"=w356, "LED1"=w355, "LED2"=w354, "LED3"=w353) -> ()  [unwired: 1 in, 1 out]
                                n111 = Equal?(x=w351, y=4.0) -> (x = y?=w350:bool)
                                n112 = Wait (ms)(milliseconds to wait=u32 100) -> ()  [unwired: 1 out]
                                }
                                }
                                }
                                n113 = Greater Or Equal?(x=w297, y=10) -> (x >= y?=w298:bool)
                                }
                              }
                              frame #1 {
                                # "RESET MYRIO"
                                n114 = call <vilib>:"Reset myRIO.vi"("error in (no error)"=errorcluster {"status"=FALSE, "code"=0, "source"=""}) -> ()  [unwired: 10 in, 1 out]
                              }
                            }
                          }
                          frame 1 {
                            # "speed"
                            # "distance"
                            # "FRONT MOVEMENT"
                            n115 = local read "Movement"() -> (w400:dbl)
                            n116 = call "front-back(SubVI).vi"("distance"=w400, "speed"=300.0) -> ()  [unwired: 10 in]
                          }
                          frame 2 {
                            # "speed"
                            # "distance"
                            # "BACK MOVEMENT"
                            n117 = local read "Movement"() -> (w405:dbl)
                            n118 = Negate(x=w405) -> (-x=w403:dbl)
                            n119 = Add(x=w403, y=10.0) -> (x+y=w404:dbl)
                            n120 = call "front-back(SubVI).vi"("distance"=w404, "speed"=150.0) -> ()  [unwired: 10 in]
                          }
                          frame 3 {
                            # "RIGTH TURN"
                            n121 = flat-sequence {
                              tunnel: [w411] -> w408
                              tunnel: w408 -> [w414]
                              tunnel: [w413] -> w407
                              tunnel: w407 -> [w434]
                              frame #0 {
                                n122 = call <vilib>:"TETRIX_Enable_DC_Controller_myRIO.vi"("Error/Flow In"=errorcluster {"status"=FALSE, "code"=0, "source"=""}) -> ("Error/Flow Out"=w412:errorcluster)  [unwired: 6 in]
                                n123 = call <vilib>:"TETRIX_Reset_Encoders_myRIO.vi"("Select Encoder"="Encoders 1 and 2", "Error/Flow In"=w412) -> ("Error/Flow Out"=w411:errorcluster)  [unwired: 5 in]
                              }
                              frame #1 {
                                n124 = while {
                                tunnel: w414 -> [w428]
                                tunnel: [w418] -> w413
                                stop <- w422 stop-if-true
                                w427 = i16 200 ("Constant Speed (Degrees per Second)")
                                # "Encoders Target"
                                # "Speed"
                                n125 = Wait Until Next ms Multiple(millisecond multiple=u32 50) -> ()  [unwired: 1 out]
                                n126 = local read "Movement"() -> (w417:dbl)
                                n127 = Subtract(x=w417, y=1.0) -> (x-y=w415:dbl)
                                n128 = Multiply(x=-11.52, y=w415) -> (x*y=w419:dbl)
                                n129 = call <vilib>:"TETRIX_Set_Motor_Target(s)_myRIO.vi"("Motor 2 Encoder Target"=w419, "Motor 1 Encoder Target"=w419, "Motor 2 Constant Speed (Degrees per Second)"=w427, "Motor 1 Contant Speed (Degrees per Second)"=w427, "Encoder Units"="Counts", "Error/Flow In"=w428) -> ("Error/Flow Out"=w430:errorcluster)  [unwired: 3 in]
                                n130 = call <vilib>:"TETRIX_Read_Motor_Busy_myRIO.vi"("Select Channel"="Motor 1", "Error/Flow In"=w430) -> ("Error/Flow Out"=w426:errorcluster, "Motor Busy?"=w424:bool)  [unwired: 4 in]
                                n131 = call <vilib>:"TETRIX_Read_Motor_Busy_myRIO.vi"("Select Channel"="Motor 2", "Error/Flow In"=w426) -> ("Error/Flow Out"=w418:errorcluster, "Motor Busy?"=w421:bool)  [unwired: 4 in]
                                n132 = And(x=w421, y=w424) -> (x .and. y?=w423:bool)
                                n133 = Not(x=w423) -> (.not. x?=w422:bool)
                                }
                              }
                              frame #2 {
                                n134 = call <vilib>:"TETRIX_Stop_Motors_myRIO.vi"("Select Channel"="Both Motors", "Error/Flow In"=w434) -> ()  [unwired: 5 in, 1 out]
                              }
                            }
                          }
                          frame 4 {
                            # "LEFT TURN"
                            n135 = flat-sequence {
                              tunnel: [w439] -> w436
                              tunnel: w436 -> [w442]
                              tunnel: [w441] -> w435
                              tunnel: w435 -> [w462]
                              frame #0 {
                                n136 = call <vilib>:"TETRIX_Enable_DC_Controller_myRIO.vi"("Error/Flow In"=errorcluster {"status"=FALSE, "code"=0, "source"=""}) -> ("Error/Flow Out"=w440:errorcluster)  [unwired: 6 in]
                                n137 = call <vilib>:"TETRIX_Reset_Encoders_myRIO.vi"("Select Encoder"="Encoders 1 and 2", "Error/Flow In"=w440) -> ("Error/Flow Out"=w439:errorcluster)  [unwired: 5 in]
                              }
                              frame #1 {
                                n138 = while {
                                tunnel: w442 -> [w456]
                                tunnel: [w450] -> w441
                                stop <- w449 stop-if-true
                                w455 = i16 200 ("Constant Speed (Degrees per Second)")
                                # "Encoders Target"
                                # "Speed"
                                n139 = Wait Until Next ms Multiple(millisecond multiple=u32 50) -> ()  [unwired: 1 out]
                                n140 = local read "Movement"() -> (w445:dbl)
                                n141 = Subtract(x=w445, y=1.0) -> (x-y=w443:dbl)
                                n142 = Multiply(x=11.55, y=w443) -> (x*y=w446:dbl)
                                n143 = call <vilib>:"TETRIX_Set_Motor_Target(s)_myRIO.vi"("Motor 2 Encoder Target"=w446, "Motor 1 Encoder Target"=w446, "Motor 2 Constant Speed (Degrees per Second)"=w455, "Motor 1 Contant Speed (Degrees per Second)"=w455, "Encoder Units"="Counts", "Error/Flow In"=w456) -> ("Error/Flow Out"=w458:errorcluster)  [unwired: 3 in]
                                n144 = call <vilib>:"TETRIX_Read_Motor_Busy_myRIO.vi"("Select Channel"="Motor 1", "Error/Flow In"=w458) -> ("Error/Flow Out"=w454:errorcluster, "Motor Busy?"=w452:bool)  [unwired: 4 in]
                                n145 = call <vilib>:"TETRIX_Read_Motor_Busy_myRIO.vi"("Select Channel"="Motor 2", "Error/Flow In"=w454) -> ("Error/Flow Out"=w450:errorcluster, "Motor Busy?"=w448:bool)  [unwired: 4 in]
                                n146 = And(x=w448, y=w452) -> (x .and. y?=w451:bool)
                                n147 = Not(x=w451) -> (.not. x?=w449:bool)
                                }
                              }
                              frame #2 {
                                n148 = call <vilib>:"TETRIX_Stop_Motors_myRIO.vi"("Select Channel"="Both Motors", "Error/Flow In"=w462) -> ()  [unwired: 5 in, 1 out]
                              }
                            }
                          }
                          frame 5 {
                            # "CALIBRATE"
                            n149 = flat-sequence {
                              frame #0 {
                                # "speed"
                                # "distance"
                                # "FRONT"
                                n150 = call "front-back(SubVI).vi"("distance"=30.0, "speed"=150.0) -> ()  [unwired: 10 in]
                              }
                              frame #1 {
                                n151 = while {
                                i -> [w467]
                                stop <- w468 stop-if-true
                                n152 = flat-sequence {
                                tunnel: [w472] -> w469
                                frame #0 {
                                n153 = Wait (ms)(milliseconds to wait=u32 100) -> ()  [unwired: 1 out]
                                }
                                frame #1 {
                                n154 = local read "hokuyo"() -> (w471:dbl[])
                                n155 = local write "hokuyo instance"(w471) -> ()
                                }
                                frame #2 {
                                n156 = local read "hokuyo instance"() -> (w473:dbl[])
                                n157 = Index Array(array=w473, index=9) -> (element=w478:dbl)
                                n158 = Index Array(array=w473, index=10) -> (element=w482:dbl)
                                n159 = Less?(x=w482, y=10.0) -> (x < y?=w481:bool)
                                n160 = Multiply(x=w478, y=2.0) -> (x*y=w484:dbl)
                                n161 = Less?(x=w478, y=400.0) -> (x < y?=w475:bool)
                                n162 = Greater?(x=w482, y=w484) -> (0:w479:bool)
                                n163 = Or(x=w481, y=w479) -> (x .or. y?=w480:bool)
                                n164 = Greater?(x=w478, y=10.0) -> (0:w476:bool)
                                n165 = And(x=w476, y=w475) -> (x .and. y?=w474:bool)
                                n166 = And(x=w474, y=w480) -> (x .and. y?=w489:bool)
                                n167 = case shown="False" w489 {
                                tunnel: w474 -> [w495 _]
                                tunnel: w482 -> [w494 _]
                                tunnel: [FALSE TRUE] -> w472
                                tunnel: w473 -> [w490 _]
                                frame False {
                                n168 = Less?(x=w494, y=400.0) -> (x < y?=w491:bool)
                                n169 = And(x=w495, y=w491) -> (x .and. y?=w493:bool)
                                n170 = case shown="False" w493 {
                                tunnel: w490 -> [w497 w505]
                                frame False {
                                # "robot is left, go right"
                                n171 = Index Array(array=w497, index=8) -> (element=w500:dbl)
                                n172 = Less?(x=w500, y=400.0) -> (x < y?=w502:bool)
                                n173 = Greater?(x=w500, y=10.0) -> (0:w499:bool)
                                n174 = And(x=w502, y=w499) -> (x .and. y?=w498:bool)
                                n175 = case shown="True" w498 {
                                frame False {
                                # "30right"
                                n176 = call "correction-right-30(SubVI).vi"() -> ()  [unwired: 12 in]
                                }
                                frame True {
                                # "15right"
                                n177 = call "correction-right-15(SubVI).vi"() -> ()  [unwired: 12 in]
                                }
                                }
                                }
                                frame True {
                                # "robot is right, go left"
                                n178 = Index Array(array=w505, index=11) -> (element=w510:dbl)
                                n179 = Less?(x=w510, y=400.0) -> (x < y?=w508:bool)
                                n180 = Greater?(x=w510, y=10.0) -> (0:w511:bool)
                                n181 = And(x=w508, y=w511) -> (x .and. y?=w512:bool)
                                n182 = case shown="True" w512 {
                                frame False {
                                # "15left"
                                n183 = call "correction-left-15(SubVI).vi"() -> ()  [unwired: 12 in]
                                }
                                frame True {
                                # "30left"
                                n184 = call "correction-left-30(SubVI).vi"() -> ()  [unwired: 12 in]
                                }
                                }
                                }
                                }
                                }
                                frame True {
                                }
                                }
                                }
                                }
                                n185 = Greater Or Equal?(x=w467, y=2) -> (x >= y?=w465:bool)
                                n186 = Or(x=w469, y=w465) -> (x .or. y?=w468:bool)
                                }
                              }
                              frame #2 {
                                n187 = flat-sequence {
                                frame #0 {
                                # "Front w/ Time"
                                n188 = call "front-time(SubVI).vi"("x"=250) -> ()  [unwired: 11 in]
                                }
                                }
                              }
                            }
                          }
                          frame 6 {
                            # "TAKE AND STORE CUBE"
                            n189 = flat-sequence {
                              tunnel: [w522] -> w517
                              tunnel: w517 -> [w530]
                              tunnel: [w527] -> w516
                              tunnel: [w541] -> w515
                              tunnel: w516 -> [w540]
                              tunnel: w515 -> [w565]
                              frame #0 {
                                # "Initialization"
                                n190 = call <vilib>:"TETRIX_Enable_Servo_Controller_myRIO.vi"("Error/Flow In"=errorcluster {"status"=FALSE, "code"=0, "source"=""}) -> ("Error/Flow Out"=w521:errorcluster)  [unwired: 6 in]
                                n191 = call <vilib>:"TETRIX_Set_Servo_Position_myRIO.vi"("Set Servo Position (0 - 180 degrees)"=u8 240, "Select Channel"="Servo 5", "Error/Flow In"=w521) -> ("Error/Flow Out"=w520:errorcluster)  [unwired: 4 in]
                                n192 = call <vilib>:"TETRIX_Set_Servo_Position_myRIO.vi"("Set Servo Position (0 - 180 degrees)"=u8 180, "Select Channel"="Servo 6", "Error/Flow In"=w520) -> ("Error/Flow Out"=w522:errorcluster)  [unwired: 4 in]
                              }
                              frame #1 {
                                n193 = while {
                                tunnel: w530 -> [w537]
                                tunnel: [w538] -> w528
                                i -> [w535]
                                stop <- w531 stop-if-true
                                n194 = call <vilib>:"TETRIX_Set_Servo_Position_myRIO.vi"("Set Servo Position (0 - 180 degrees)"=u8 180, "Select Channel"="Servo 4", "Error/Flow In"=w537) -> ("Error/Flow Out"=w538:errorcluster)  [unwired: 4 in]
                                n195 = Equal?(x=230, y=w535) -> (x = y?=w531:bool)
                                n196 = Wait (ms)(milliseconds to wait=u32 10) -> ()  [unwired: 1 out]
                                }
                                n197 = call <vilib>:"TETRIX_Set_Servo_Position_myRIO.vi"("Set Servo Position (0 - 180 degrees)"=u8 90, "Select Channel"="Servo 4", "Error/Flow In"=w528) -> ("Error/Flow Out"=w527:errorcluster)  [unwired: 4 in]
                              }
                              frame #2 {
                                n198 = while {
                                shift-right: [w555] -> w542
                                shift-left: w540 -> [w553]
                                i -> [w550]
                                stop <- w548 stop-if-true
                                # "Delay"
                                n199 = Equal?(x=w550, y=60) -> (x = y?=w547:bool)
                                n200 = case shown="True" w547 {
                                tunnel: [FALSE w557] -> w548
                                frame False {
                                }
                                frame True {
                                n201 = while {
                                shift-right: [w558] -> w557
                                shift-left: _ -> [_]
                                tunnel: [w559] -> _
                                i -> [w560]
                                stop <- w558 stop-if-true
                                n202 = call <vilib>:"TETRIX_Set_Servo_Position_myRIO.vi"("Set Servo Position (0 - 180 degrees)"=u8 0, "Select Channel"="Servo 4") -> ("Error/Flow Out"=w559:errorcluster)  [unwired: 5 in]
                                n203 = Wait (ms)(milliseconds to wait=u32 10) -> ()  [unwired: 1 out]
                                n204 = Equal?(x=230, y=w560) -> (x = y?=w558:bool)
                                }
                                }
                                }
                                n205 = call <vilib>:"TETRIX_Set_Servo_Position_myRIO.vi"("Set Servo Position (0 - 180 degrees)"=u8 120, "Select Channel"="Servo 5", "Error/Flow In"=w553) -> ("Error/Flow Out"=w555:errorcluster)  [unwired: 4 in]
                                n206 = Wait (ms)(milliseconds to wait=u32 10) -> ()  [unwired: 1 out]
                                }
                                n207 = for {
                                N: 20 -> [_]
                                shift-right: [w544] -> w541
                                shift-left: w542 -> [w545]
                                n208 = call <vilib>:"TETRIX_Set_Servo_Position_myRIO.vi"("Set Servo Position (0 - 180 degrees)"=u8 180, "Select Channel"="Servo 5", "Error/Flow In"=w545) -> ("Error/Flow Out"=w544:errorcluster)  [unwired: 4 in]
                                }
                              }
                              frame #3 {
                                n209 = call <vilib>:"TETRIX_Reset_Servo_Controller_myRIO.vi"("Error/Flow In"=w565) -> ()  [unwired: 6 in, 1 out]
                              }
                            }
                          }
                          frame 7 {
                            # "TAKE AND HOLD CUBE"
                            n210 = flat-sequence {
                              tunnel: [w573] -> w568
                              tunnel: w568 -> [w581]
                              tunnel: [w578] -> w567
                              tunnel: w567 -> [w595]
                              tunnel: [w590] -> w566
                              tunnel: w566 -> [w622]
                              frame #0 {
                                # "Initialization"
                                n211 = call <vilib>:"TETRIX_Enable_Servo_Controller_myRIO.vi"("Error/Flow In"=errorcluster {"status"=FALSE, "code"=0, "source"=""}) -> ("Error/Flow Out"=w572:errorcluster)  [unwired: 6 in]
                                n212 = call <vilib>:"TETRIX_Set_Servo_Position_myRIO.vi"("Set Servo Position (0 - 180 degrees)"=u8 250, "Select Channel"="Servo 5", "Error/Flow In"=w572) -> ("Error/Flow Out"=w571:errorcluster)  [unwired: 4 in]
                                n213 = call <vilib>:"TETRIX_Set_Servo_Position_myRIO.vi"("Set Servo Position (0 - 180 degrees)"=u8 180, "Select Channel"="Servo 6", "Error/Flow In"=w571) -> ("Error/Flow Out"=w573:errorcluster)  [unwired: 4 in]
                              }
                              frame #1 {
                                n214 = while {
                                tunnel: w581 -> [w588]
                                tunnel: [w589] -> w579
                                i -> [w586]
                                stop <- w582 stop-if-true
                                n215 = call <vilib>:"TETRIX_Set_Servo_Position_myRIO.vi"("Set Servo Position (0 - 180 degrees)"=u8 180, "Select Channel"="Servo 4", "Error/Flow In"=w588) -> ("Error/Flow Out"=w589:errorcluster)  [unwired: 4 in]
                                n216 = Equal?(x=250, y=w586) -> (x = y?=w582:bool)
                                n217 = Wait (ms)(milliseconds to wait=u32 10) -> ()  [unwired: 1 out]
                                }
                                n218 = call <vilib>:"TETRIX_Set_Servo_Position_myRIO.vi"("Set Servo Position (0 - 180 degrees)"=u8 90, "Select Channel"="Servo 4", "Error/Flow In"=w579) -> ("Error/Flow Out"=w578:errorcluster)  [unwired: 4 in]
                              }
                              frame #2 {
                                n219 = while {
                                shift-right: [w612] -> w591
                                shift-left: w595 -> [w610]
                                i -> [w607]
                                stop <- w605 stop-if-true
                                # "Delay"
                                n220 = Equal?(x=w607, y=60) -> (x = y?=w604:bool)
                                n221 = case shown="True" w604 {
                                tunnel: [FALSE w614] -> w605
                                frame False {
                                }
                                frame True {
                                n222 = while {
                                shift-right: [w615] -> w614
                                shift-left: _ -> [_]
                                tunnel: [w616] -> _
                                i -> [w617]
                                stop <- w615 stop-if-true
                                n223 = call <vilib>:"TETRIX_Set_Servo_Position_myRIO.vi"("Set Servo Position (0 - 180 degrees)"=u8 0, "Select Channel"="Servo 4") -> ("Error/Flow Out"=w616:errorcluster)  [unwired: 5 in]
                                n224 = Wait (ms)(milliseconds to wait=u32 10) -> ()  [unwired: 1 out]
                                n225 = Equal?(x=60, y=w617) -> (x = y?=w615:bool)
                                }
                                }
                                }
                                n226 = call <vilib>:"TETRIX_Set_Servo_Position_myRIO.vi"("Set Servo Position (0 - 180 degrees)"=u8 120, "Select Channel"="Servo 5", "Error/Flow In"=w610) -> ("Error/Flow Out"=w612:errorcluster)  [unwired: 4 in]
                                n227 = Wait (ms)(milliseconds to wait=u32 10) -> ()  [unwired: 1 out]
                                }
                                n228 = for {
                                N: 20 -> [_]
                                shift-right: [w601] -> w592
                                shift-left: w591 -> [w600]
                                n229 = call <vilib>:"TETRIX_Set_Servo_Position_myRIO.vi"("Set Servo Position (0 - 180 degrees)"=u8 90, "Select Channel"="Servo 5", "Error/Flow In"=w600) -> ("Error/Flow Out"=w601:errorcluster)  [unwired: 4 in]
                                }
                                n230 = for {
                                N: 50 -> [_]
                                shift-right: [w596] -> w590
                                shift-left: w592 -> [w597]
                                n231 = call <vilib>:"TETRIX_Set_Servo_Position_myRIO.vi"("Set Servo Position (0 - 180 degrees)"=u8 85, "Select Channel"="Servo 6", "Error/Flow In"=w597) -> ("Error/Flow Out"=w596:errorcluster)  [unwired: 4 in]
                                }
                              }
                              frame #3 {
                                n232 = call <vilib>:"TETRIX_Reset_Servo_Controller_myRIO.vi"("Error/Flow In"=w622) -> ()  [unwired: 6 in, 1 out]
                              }
                            }
                          }
                          frame 8 {
                            # "PLACE CUBE"
                            n233 = flat-sequence {
                              tunnel: [w629] -> w628
                              tunnel: [w639] -> w627
                              tunnel: w628 -> [w637]
                              tunnel: w627 -> [w646]
                              tunnel: [w644] -> w626
                              tunnel: [w653] -> w625
                              tunnel: w626 -> [w651]
                              tunnel: [w660] -> w624
                              tunnel: w625 -> [w658]
                              tunnel: w624 -> [w672]
                              tunnel: [w671] -> w623
                              tunnel: w623 -> [w691]
                              frame #0 {
                                # "Open claw a bit"
                                # "Initialization"
                                n234 = call <vilib>:"TETRIX_Enable_Servo_Controller_myRIO.vi"("Error/Flow In"=errorcluster {"status"=FALSE, "code"=0, "source"=""}) -> ("Error/Flow Out"=w633:errorcluster)  [unwired: 6 in]
                                n235 = call <vilib>:"TETRIX_Set_Servo_Position_myRIO.vi"("Set Servo Position (0 - 180 degrees)"=u8 140, "Select Channel"="Servo 5", "Error/Flow In"=w633) -> ("Error/Flow Out"=w632:errorcluster)  [unwired: 4 in]
                                n236 = call <vilib>:"TETRIX_Set_Servo_Position_myRIO.vi"("Set Servo Position (0 - 180 degrees)"=u8 90, "Select Channel"="Servo 6", "Error/Flow In"=w632) -> ("Error/Flow Out"=w629:errorcluster)  [unwired: 4 in]
                              }
                              frame #1 {
                                # "Lift up a bit"
                                n237 = for {
                                N: 50 -> [_]
                                shift-right: [w640] -> w639
                                shift-left: w637 -> [w641]
                                n238 = call <vilib>:"TETRIX_Set_Servo_Position_myRIO.vi"("Set Servo Position (0 - 180 degrees)"=u8 70, "Select Channel"="Servo 6", "Error/Flow In"=w641) -> ("Error/Flow Out"=w640:errorcluster)  [unwired: 4 in]
                                }
                              }
                              frame #2 {
                                # "Close claw"
                                n239 = for {
                                N: 20 -> [_]
                                shift-right: [w647] -> w644
                                shift-left: w646 -> [w648]
                                n240 = call <vilib>:"TETRIX_Set_Servo_Position_myRIO.vi"("Set Servo Position (0 - 180 degrees)"=u8 120, "Select Channel"="Servo 5", "Error/Flow In"=w648) -> ("Error/Flow Out"=w647:errorcluster)  [unwired: 4 in]
                                }
                              }
                              frame #3 {
                                # "Lift down"
                                n241 = for {
                                N: 50 -> [_]
                                shift-right: [w654] -> w653
                                shift-left: w651 -> [w655]
                                n242 = call <vilib>:"TETRIX_Set_Servo_Position_myRIO.vi"("Set Servo Position (0 - 180 degrees)"=u8 180, "Select Channel"="Servo 6", "Error/Flow In"=w655) -> ("Error/Flow Out"=w654:errorcluster)  [unwired: 4 in]
                                }
                              }
                              frame #4 {
                                n243 = while {
                                tunnel: w658 -> [w670]
                                tunnel: [w663] -> w661
                                i -> [w668]
                                stop <- w664 stop-if-true
                                # "Claw full extend"
                                n244 = call <vilib>:"TETRIX_Set_Servo_Position_myRIO.vi"("Set Servo Position (0 - 180 degrees)"=u8 180, "Select Channel"="Servo 4", "Error/Flow In"=w670) -> ("Error/Flow Out"=w663:errorcluster)  [unwired: 4 in]
                                n245 = Equal?(x=170, y=w668) -> (x = y?=w664:bool)
                                n246 = Wait (ms)(milliseconds to wait=u32 10) -> ()  [unwired: 1 out]
                                }
                                n247 = call <vilib>:"TETRIX_Set_Servo_Position_myRIO.vi"("Set Servo Position (0 - 180 degrees)"=u8 0, "Select Channel"="Servo 4", "Error/Flow In"=w661) -> ("Error/Flow Out"=w660:errorcluster)  [unwired: 4 in]
                              }
                              frame #5 {
                                n248 = while {
                                shift-right: [w681] -> w671
                                shift-left: w672 -> [w679]
                                i -> [w676]
                                stop <- w674 stop-if-true
                                # "Open claw and go back to initial position"
                                # "Delay"
                                n249 = Equal?(x=w676, y=60) -> (x = y?=w673:bool)
                                n250 = case shown="True" w673 {
                                tunnel: [FALSE w683] -> w674
                                frame False {
                                }
                                frame True {
                                n251 = while {
                                shift-right: [w684] -> w683
                                shift-left: _ -> [_]
                                tunnel: [w685] -> _
                                i -> [w686]
                                stop <- w684 stop-if-true
                                n252 = Equal?(x=230, y=w686) -> (x = y?=w684:bool)
                                n253 = call <vilib>:"TETRIX_Set_Servo_Position_myRIO.vi"("Set Servo Position (0 - 180 degrees)"=u8 0, "Select Channel"="Servo 4") -> ("Error/Flow Out"=w685:errorcluster)  [unwired: 5 in]
                                n254 = Wait (ms)(milliseconds to wait=u32 10) -> ()  [unwired: 1 out]
                                }
                                }
                                }
                                n255 = call <vilib>:"TETRIX_Set_Servo_Position_myRIO.vi"("Set Servo Position (0 - 180 degrees)"=u8 180, "Select Channel"="Servo 5", "Error/Flow In"=w679) -> ("Error/Flow Out"=w681:errorcluster)  [unwired: 4 in]
                                n256 = Wait (ms)(milliseconds to wait=u32 10) -> ()  [unwired: 1 out]
                                }
                              }
                              frame #6 {
                                n257 = call <vilib>:"TETRIX_Reset_Servo_Controller_myRIO.vi"("Error/Flow In"=w691) -> ()  [unwired: 6 in, 1 out]
                              }
                            }
                          }
                          frame 9 {
                            # "CHECK COLOR"
                            n258 = flat-sequence {
                              tunnel: [w731] -> w703
                              tunnel: [w720] -> w702
                              tunnel: [w712] -> w701
                              tunnel: [w712] -> w700
                              tunnel: [w720] -> w699
                              tunnel: w703 -> [w765]
                              tunnel: [w765] -> w698
                              tunnel: w702 -> [w761]
                              tunnel: [w760] -> w697
                              tunnel: w701 -> [w758]
                              tunnel: [w759] -> w696
                              tunnel: w700 -> [w750]
                              tunnel: [w752] -> w695
                              tunnel: [w751] -> w694
                              tunnel: w699 -> [w749]
                              tunnel: w698 -> [w783]
                              tunnel: [w783] -> w693
                              tunnel: w697 -> [w775]
                              tunnel: [w776] -> w692
                              tunnel: w696 -> [w774]
                              tunnel: w695 -> [w767]
                              tunnel: w694 -> [w766]
                              tunnel: w693 -> [w786]
                              tunnel: w692 -> [w785]
                              frame #0 {
                                "Box Green" <- -1.0 ("Green")
                                "Box Red" <- -1.0 ("Red")
                                "Box Blue" <- -1.0 ("Blue")
                                "Cube Green" <- -1.0 ("Green")
                                "Cube Red" <- -1.0 ("Red")
                                "Cube Blue" <- -1.0 ("Blue")
                                "COLOR BOX" <- 15.0 ("COLOR BOX")
                                "COLOR CUBE" <- 15.0 ("COLOR CUBE")
                              }
                              frame #1 {
                                w736 = T16 4 items=["Grayscale (U8)", "Grayscale (I16)", "Grayscale (SGL)", "Complex (CSG)", "RGB (U32)", "HSL (U32)", "RGB (U64)", "Grayscale (U16)"] ("Image Type")
                                n259 = call <vilib>:"IMAQdx Open Camera.vi"("Camera Control Mode"=IMAQdx_Camera_Control_Mode."Controller", "Session In"=T10 "cam3") -> ("error out"=w741:errorcluster, "Session Out"=w740:T10)  [unwired: 8 in]
                                n260 = call "IMAQ Create"("Image Name"="untitled", "Image Type"=w736) -> ("New Image"=w734:T1)  [unwired: 3 in, 1 out]
                                n261 = Format Date/Time String(time format string (%c)="%H-%M-%S") -> (date/time string=w719:string)  [unwired: 2 in]
                                n262 = Build Array(250.0 ("element"), 400.0 ("element"), 300.0 ("element"), 450.0 ("element")) -> (→"Cube Array":dbl[])
                                n263 = Build Array(220.0 ("element"), 190.0 ("element"), 270.0 ("element"), 240.0 ("element")) -> (→"Box Array":dbl[])
                                n264 = call <vilib>:"IMAQdx Configure Grab.vi"("error in"=w741, "Session In"=w740) -> ("error out"=w733:errorcluster, "Session Out"=w739:T10)  [unwired: 8 in]
                                n265 = Concatenate Strings("/home/lvuser/images-log/color_" ("string"), w719) -> (w717:string)
                                n266 = for {
                                N: 5 -> [_]
                                shift-right: [w747] -> w731
                                shift-left: w739 -> [w748]
                                shift-right: [w743] -> w712
                                shift-left: w734 -> [w745]
                                shift-right: [w746] -> w720
                                shift-left: w733 -> [w744]
                                n267 = call <vilib>:"IMAQdx Snap2.vi"("error in"=w744, "Image In"=w745, "Session In"=w748) -> ("error out"=w746:errorcluster, "Image Out"=w743:T1, "Session Out"=w747:T10)  [unwired: 6 in]
                                n268 = Wait Until Next ms Multiple(millisecond multiple=u32 250) -> ()  [unwired: 1 out]
                                }
                                "Color Footage" <- w712
                                n269 = Concatenate Strings(w717, ".jpg" ("string")) -> (w714:string)
                                n270 = String To Path(string=w714) -> (path=w713:path)
                                n271 = call-poly "IMAQ Write File 2"("error in (no error)"=w720, "File Path"=w713, "Image"=w712) -> ()  [unwired: 7 in, 2 out]
                              }
                              frame #2 {
                                w753 = T16 4 items=["Grayscale (U8)", "Grayscale (I16)", "Grayscale (SGL)", "Complex (CSG)", "RGB (U32)", "HSL (U32)", "RGB (U64)", "Grayscale (U16)"] ("Image Type")
                                w764 = T16 4 items=["Grayscale (U8)", "Grayscale (I16)", "Grayscale (SGL)", "Complex (CSG)", "RGB (U32)", "HSL (U32)", "RGB (U64)", "Grayscale (U16)"] ("Image Type")
                                n272 = call "IMAQ Create"("Image Name"="Box Crop", "Image Type"=w764) -> ("New Image"=w763:T1)  [unwired: 3 in, 1 out]
                                n273 = call "IMAQ Create"("Image Name"="Cube Crop", "Image Type"=w753) -> ("New Image"=w754:T1)  [unwired: 3 in, 1 out]
                                n274 = local read "Cube Array"() -> (w756:dbl[])
                                n275 = local read "Box Array"() -> (w757:dbl[])
                                n276 = call "IMAQ Extract"("Optional Rectangle"=w757, "error in (no error)"=w761, "Image Dst"=w763, "Image Src"=w758) -> ("error out"=w760:errorcluster, "Image Dst Out"=w759:T1)  [unwired: 6 in]
                                n277 = call "IMAQ Extract"("Optional Rectangle"=w756, "error in (no error)"=w749, "Image Dst"=w754, "Image Src"=w750) -> ("error out"=w752:errorcluster, "Image Dst Out"=w751:T1)  [unwired: 6 in]
                              }
                              frame #3 {
                                n278 = call "IMAQ ColorHistogram"("Image Src"=w766, "error in (no error)"=w767) -> ("Red or Hue or X or L* Histogram Report"=w773:T21, "Green or Sat or Y or a* Histogram Report"=w771:T21, "Blue or Luma or Val or Inten or Z or b* Histogram Report"=w770:T21)  [unwired: 4 in, 1 out]
                                n279 = call "IMAQ ColorHistogram"("Image Src"=w774, "error in (no error)"=w775) -> ("Red or Hue or X or L* Histogram Report"=w777:T21, "Green or Sat or Y or a* Histogram Report"=w779:T21, "Blue or Luma or Val or Inten or Z or b* Histogram Report"=w780:T21, "error out"=w776:errorcluster)  [unwired: 4 in]
                                n280 = Unbundle By Name(w773) -> ("Mean Value"=w772:sgl)
                                n281 = Unbundle By Name(w770) -> ("Mean Value"=w769:sgl)
                                n282 = Unbundle By Name(w771) -> ("Mean Value"=w768:sgl)
                                n283 = Unbundle By Name(w777) -> ("Mean Value"=w778:sgl)
                                n284 = Unbundle By Name(w780) -> ("Mean Value"=w781:sgl)
                                n285 = Unbundle By Name(w779) -> ("Mean Value"=w782:sgl)
                                n286 = local write "Cube Green"(w768) -> ()
                                n287 = local write "Cube Blue"(w769) -> ()
                                n288 = local write "Cube Red"(w772) -> ()
                                n289 = local write "Box Green"(w782) -> ()
                                n290 = local write "Box Blue"(w781) -> ()
                                n291 = local write "Box Red"(w778) -> ()
                              }
                              frame #4 {
                                n292 = call <vilib>:"IMAQdx Close Camera.vi"("error in"=w785, "Session In"=w786) -> ()  [unwired: 9 in, 1 out]
                                n293 = Wait (ms)(milliseconds to wait=u32 100) -> ()  [unwired: 1 out]
                              }
                              frame #5 {
                                # "Color Detection Algorithm"
                                n294 = local read "Box Red"() -> (w790:dbl)
                                n295 = local read "Box Green"() -> (w794:dbl)
                                n296 = local read "Box Blue"() -> (w793:dbl)
                                n297 = local read "Cube Red"() -> (w792:dbl)
                                n298 = local read "Cube Green"() -> (w791:dbl)
                                n299 = local read "Cube Blue"() -> (w789:dbl)
                                n300 = call "color-detection(SubVI).vi"("Cube Blue"=w789, "Cube Green"=w791, "Box Red"=w790, "Cube Red"=w792, "Box Blue"=w793, "Box Green"=w794) -> ("COLOR CUBE"=w787:dbl, "COLOR BOX"=w788:dbl)  [unwired: 4 in]
                                n301 = local write "COLOR CUBE"(w787) -> ()
                                n302 = local write "COLOR BOX"(w788) -> ()
                              }
                              frame #6 {
                                n303 = local read "COLOR CUBE"() -> (w801:dbl)
                                n304 = local read "COLOR BOX"() -> (w800:dbl)
                                n305 = local read "Colors String"() -> (w797:string)
                                n306 = Number To Decimal String(number=w801) -> (decimal integer string=w805:string)  [unwired: 1 in]
                                n307 = Number To Decimal String(number=w800) -> (decimal integer string=w802:string)  [unwired: 1 in]
                                n308 = Concatenate Strings(w805, "," ("string")) -> (w803:string)
                                n309 = Concatenate Strings(w803, w802) -> (w798:string)
                                n310 = Concatenate Strings(w798, "," ("string")) -> (w796:string)
                                n311 = Concatenate Strings(w797, w796) -> (w795:string)
                                n312 = local write "Colors String"(w795) -> ()
                              }
                              frame #7 {
                                # "10 BLUE\n11 GREEN\n12 YELLOW\n13 RED\n14 ORANGE\n15 UNKNOWN"
                                # "Write Colors File"
                                n313 = local read "Colors String"() -> (w809:string)
                                n314 = String Length(string=w809) -> (length=w807:i32)
                                n315 = Equal?(x=w807, y=18) -> (x = y?=w806:bool)
                                n316 = case shown="True" w806 {
                                tunnel: w809 -> [w810 w824]
                                frame False {
                                n317 = String Length(string=w810) -> (length=w813:i32)
                                n318 = Equal?(x=w813, y=24) -> (x = y?=w811:bool)
                                n319 = case shown="True" w811 {
                                frame False {
                                }
                                frame True {
                                n320 = local read "COLOR BOX"() -> (w816:dbl)
                                n321 = local read "COLOR CUBE"() -> (w815:dbl)
                                n322 = Number To Decimal String(number=w816) -> (decimal integer string=w821:string)  [unwired: 1 in]
                                n323 = Number To Decimal String(number=w815) -> (decimal integer string=w817:string)  [unwired: 1 in]
                                n324 = Concatenate Strings(w817, "," ("string")) -> (w820:string)
                                n325 = Concatenate Strings(w820, w821) -> (w822:string)
                                n326 = Concatenate Strings(w822, "," ("string")) -> (w814:string)
                                n327 = Write to Text File(file (use dialog)=path "/home/lvuser/cubes4Colors.txt", text=w814) -> ()  [unwired: 2 in, 3 out]
                                }
                                }
                                }
                                frame True {
                                n328 = flat-sequence {
                                tunnel: path "/home/lvuser/cubes3Colors.txt" ("file (use dialog)") -> [w827]
                                tunnel: w824 -> [w828]
                                tunnel: [w829] -> w825
                                tunnel: w825 -> [w838]
                                frame #0 {
                                n329 = Write to Text File(file (use dialog)=w827, text=w828) -> ()  [unwired: 2 in, 3 out]
                                }
                                frame #1 {
                                n330 = while {
                                tunnel: [w830] -> w829
                                stop <- w831 stop-if-true
                                w830 = path "/home/lvuser/cubes3Flag.txt" ("file (use dialog)")
                                n331 = call <vilib>:"Check if File or Folder Exists.vi"("path"=w830) -> ("file or folder exists?"=w831:bool)  [unwired: 8 in, 2 out]
                                n332 = Wait (ms)(milliseconds to wait=u32 500) -> ()  [unwired: 1 out]
                                }
                                }
                                frame #2 {
                                n333 = Read from Text File(file (use dialog)=w838) -> (text=w836:string)  [unwired: 3 in, 3 out]
                                n334 = String Subset(string=w836, length (rest)=1 ("length (rest)")) -> (substring=w834:string)  [unwired: 1 in]
                                n335 = Equal?(x=w834, y="1") -> (x = y?=w833:bool)
                                n336 = local write "Cubes 3 Flag"(w833) -> ()
                                }
                                }
                                }
                                }
                              }
                            }
                          }
                          frame 10 {
                            # "speed"
                            # "distance"
                            # "FRONT"
                            # "PARKING"
                            n337 = local read "Movement"() -> (w839:dbl)
                            n338 = call "front-back(SubVI).vi"("distance"=w839, "speed"=100.0) -> ()  [unwired: 10 in]
                          }
                          frame 15 {
                            # "APROACH CUBE WITHOUT CALIBRATION"
                            # "Front w/ Time"
                            n339 = call "front-time(SubVI).vi"("x"=350) -> ()  [unwired: 11 in]
                          }
                        }
                      }
                    }
                  }
                }
              }
              n340 = local read "Cubes 3 Flag"() -> (w267:bool)
            }
          }
          frame #4 {
            n341 = while {
              stop <- w842 stop-if-true
              n342 = Wait (ms)(milliseconds to wait=u32 500) -> ()  [unwired: 1 out]
              n343 = call <vilib>:"Check if File or Folder Exists.vi"("path"=path "/home/lvuser/route2.csv" ("file (use dialog)")) -> ("file or folder exists?"=w842:bool)  [unwired: 8 in, 2 out]
              n344 = Not(x=w842) -> (.not. x?=w843:bool)
              n345 = local write "CHECK route2.csv"(w842) -> ()
              n346 = local write "Cubes 3 Flag"(w843) -> ()
            }
          }
        }
      }
    }
    frame #12 {
      n347 = local read "Algorithm log"() -> (w846:string)
      n348 = Write to Text File(file (use dialog)=path "/home/lvuser/labview.log", text=w846) -> ()  [unwired: 2 in, 3 out]
    }
  }
  n349 = while {
    tunnel: [w848] -> w3
    stop <- w848 stop-if-true
    n350 = local read "Hokuyo Init"() -> (w848:bool)
  }
  n351 = case shown="True" w3 {
    frame False {
    }
    frame True {
      w853 = u32 2 items=["Convert to Latest", "SCIP 1.1", "SCIP 2.0"] ("Protocol")
      n352 = Initialize Array(0.0 ("element"), 10 ("dimension size")) -> (→"hokuyo" →"hokuyo instance":dbl[])
      n353 = call-poly <instrlib>:"Initialize.vi"("Reset? (F: No)"=FALSE ("Reset Instrument (Disabled)"), "Checksum (Disabled)"=FALSE ("Checksum"), "ID Query? (Enabled)"=TRUE ("ID Query?"), "Protocol (2: SCIP 2.0)"=w853, "VISA resource name"="USB0::0x15D1::0x0000::NI-VISA-1005::1::RAW") -> ("error out"=w856:errorcluster, "VISA resource name out"=w857:refnum<visa-resource-name>)  [unwired: 5 in]
      n354 = while {
        tunnel: w857 -> [w867]
        tunnel: w856 -> [w866]
        stop <- FALSE stop-if-true
        w863 = u16 3 items=["2 Byte"=2, "3 Byte"=3] ("Encoding Width")
        n355 = call <instrlib>:"Acquire Data.vi"("Data Encoding Width (3 Byte)"=w863, "Cluster Count (1)"=20.0 ("Cluster Count"), "error in (no error)"=w866, "End Point (120°)"=40.0 ("End Point"), "Start Point (-120°)"=-60.0 ("Start Point"), "VISA resource name"=w867) -> ("error out"=w864:errorcluster, "Magnitude"=w865:dbl[])  [unwired: 2 in, 2 out]
        n356 = case shown="Error" w864 {
          selector: w864 -> [_ w869]
          tunnel: w865 -> [w868 _]
          frame No Error {
            n357 = local write "hokuyo"(w868) -> ()
          }
          frame Error {
            "?" <- w869
          }
        }
      }
    }
  }
  n358 = while {
    tunnel: [w870] -> w2
    stop <- w870 stop-if-true
    n359 = local read "Delete Files"() -> (w870:bool)
  }
  n360 = case shown="True" w2 {
    frame False {
    }
    frame True {
      n361 = call <vilib>:"System Exec.vi"("expected output size  (4096)"=u32 1, "run minimized? (F)"=FALSE, "wait until completion? (T)"=TRUE, "command line"="/home/lvuser/cleanup.sh") -> ("return code"=→"RETURN VALUE":i32, "standard error"=→"STD ERROR":string, "standard output"=→"TERMINAL OUTPUT":string)  [unwired: 4 in, 1 out]
    }
  }
  n362 = while {
    tunnel: [w878] -> w1
    stop <- w878 stop-if-true
    n363 = local read "START ALGO"() -> (w878:bool)
  }
  n364 = case shown="True" w1 {
    frame False {
    }
    frame True {
      n365 = call <vilib>:"System Exec.vi"("expected output size  (4096)"=u32 1, "run minimized? (F)"=TRUE, "wait until completion? (T)"=FALSE, "command line"="/home/lvuser/algorithm.sh") -> ("return code"=w880:i32, "standard error"=w881:string, "standard output"=→"Algorithm log":string)  [unwired: 4 in, 1 out]
      n366 = local write "RETURN VALUE"(w880) -> ()
      n367 = local write "STD ERROR"(w881) -> ()
    }
  }
